vi "Init.vi"(7 "Error Checking (Full)":T1=enum."Full", 8 "error in (no error)":errorcluster, 10 "DeviceComms":refnum<class "DeviceComms.lvclass">) -> (0 "error out":errorcluster, 2 "Identity":T2, 3 "Session out":refnum<class "Session.lvclass">)   [LabVIEW 2020, in "CTI.lvlib" / "Session.lvclass"]
uses:
  Session.lvclass
  DeviceComms/DeviceComms.lvclass
  Identity.ctl
  Error Reporting.ctl
  Resources.ctl
  GPIO Number.ctl
  GPIO/GPIO.lvclass
  ADC Number.ctl
  AI/AI.lvclass
  PWM/PWM.lvclass
  UART Number.ctl
  UART/UART.lvclass
  I2C Number.ctl
  I2C/I2C.lvclass
  SPI Number.ctl
  SPI/SPI.lvclass
  Session.lvclass/Session.ctl
  CTI.lvlib
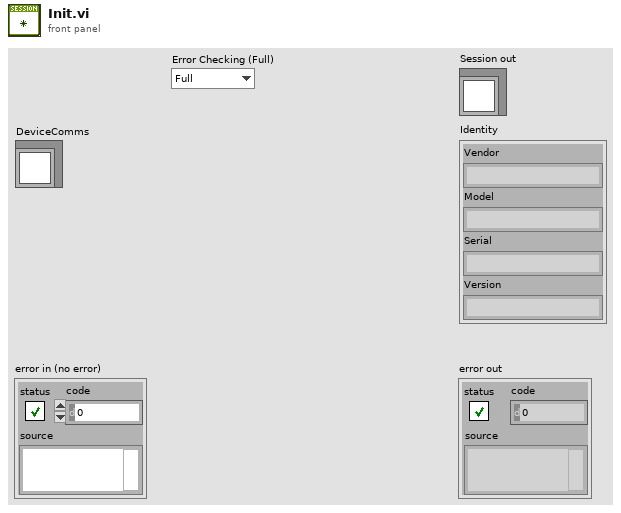
[diagram p1: front panel]
types:
  T1 = typedef "CTI.lvlib/Error Reporting.ctl" = enum16{"Minimal", "Moderate", "Full"}
  T2 = typedef "CTI.lvlib/Identity.ctl" = cluster{"Vendor":string, "Model":string, "Serial":string, "Version":string}
  T3 = typedef "CTI.lvlib/Session.lvclass/Resources.ctl" = cluster{"GPIO":map{T4, refnum<class "GPIO.lvclass">}, "AI":map{T5, refnum<class "AI.lvclass">}, "PWM":map{T4, refnum<class "PWM.lvclass">}, "UART":map{T6, refnum<class "UART.lvclass">}, "I2C":map{T7, refnum<class "I2C.lvclass">}, "SPI":map{T8, refnum<class "SPI.lvclass">}}
  T4 = typedef "CTI.lvlib/GPIO Number.ctl" = i8
  T5 = typedef "CTI.lvlib/ADC Number.ctl" = i8
  T6 = typedef "CTI.lvlib/UART Number.ctl" = i8
  T7 = typedef "CTI.lvlib/I2C Number.ctl" = i8
  T8 = typedef "CTI.lvlib/SPI Number.ctl" = i8
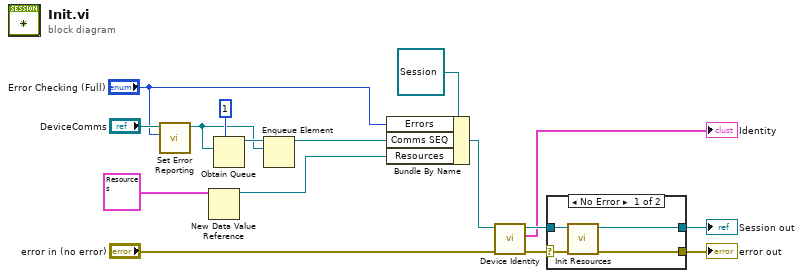
[diagram p0: block diagram]
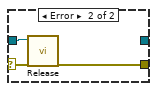
[diagram p2: hidden frame]
diagram:
  n1 = call-dynamic "Set Error Reporting.vi"("Error Reporting"="Error Checking (Full)", "DeviceComms in"="DeviceComms") -> ("DeviceComms out"=w2:refnum<class "DeviceComms.lvclass">)  [unwired: 8 in, 1 out]
  n2 = New Data Value Reference(data value=T3 {"GPIO"={}, "AI"={}, "PWM"={}, "UART"={}, "I2C"={}, "SPI"={}} ("Resources")) -> (data value reference=w3:refnum<data-value>)  [unwired: 1 in, 1 out]
  n3 = Obtain Queue(max queue size (-1, unlimited)=1, element data type=w2) -> (queue out=w15:refnum<queue>)  [unwired: 3 in, 2 out]
  n4 = Enqueue Element(queue=w15, element=w2) -> (queue out=w13:refnum<queue>)  [unwired: 2 in, 2 out]
  n5 = Bundle By Name(cluster=refnum<class "Session.lvclass"> refnum ("Session in"), "Errors"="Error Checking (Full)", "Comms SEQ"=w13, "Resources"=w3) -> (w11:refnum<class "Session.lvclass">)
  n6 = call "Device Identity.vi"("error in (no error)"="error in (no error)", "Session in"=w11) -> ("error out"=w9:errorcluster, "Identity"=→"Identity":T2, "Session out"=w8:refnum<class "Session.lvclass">)  [unwired: 7 in]
  n7 = case shown="No Error" w9 {
    selector: w9 -> [w20 w22]
    tunnel: w8 -> [w18 w21]
    tunnel: [w17 _] -> w7
    tunnel: [w19 w22] -> w6
    frame No Error {
      n8 = call "Init Resources.vi"("error in (no error)"=w20, "Session in"=w18) -> ("error out"=w19:errorcluster, "Session out"=w17:refnum<class "Session.lvclass">)  [unwired: 8 in]
    }
    frame Error {
      n9 = call-dynamic "Release.vi"("Session in"=w21) -> ()  [unwired: 10 in, 1 out]
    }
  }
  "error out" <- w6
  "Session out" <- w7
